vi "set_ref_clus_LakeShore218.vi"(6 "cluster_ref":T1, 10 "value_array":dbl[](array[numeric])=[0.0, 0.0, 0.0, 0.0, 0.0, 0.0, 0.0, 0.0], 11 "status":bool) -> ()   [LabVIEW 2019]
uses:
  cluster_ref_LakeShore218.ctl
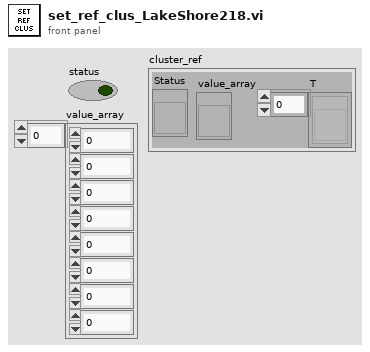
[diagram p1: front panel]
types:
  T1 = typedef "cluster_ref_LakeShore218.ctl" = cluster{"Status":refnum<vi>, "value_array":refnum<vi>, "T":refnum<vi>[]}
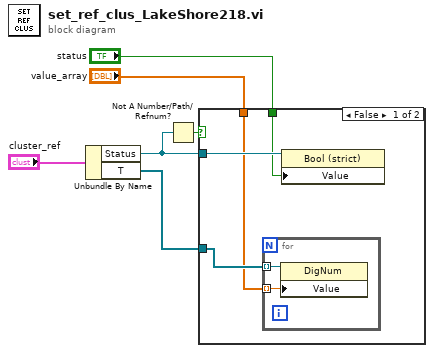
[diagram p0: block diagram]
diagram:
  n1 = Unbundle By Name("cluster_ref") -> ("Status"=w5:refnum<vi>, "T"=w1:refnum<vi>[])
  n2 = Not A Number/Path/Refnum?(number/path/refnum=w5) -> (NaN/Path/Refnum?=w6:bool)
  n3 = case shown="False" w6 {
    tunnel: w5 -> [w10 _]
    tunnel: "status" -> [w9 _]
    tunnel: "value_array" -> [w7 _]
    tunnel: w1 -> [w8 _]
    frame False {
      n4 = for {
        tunnel: w8 -> [w12] mode=indexing
        tunnel: w7 -> [w11] mode=indexing
        n5 = property class="DigNum"(reference=w12, "Value"=w11) -> ()  [unwired: 1 in, 2 out]
      }
      n6 = property class="Bool (strict)"(reference=w10, "Value"=w9) -> ()  [unwired: 1 in, 2 out]
    }
    frame True {
    }
  }
